vi "Test Communication.vi"() -> ()   [LabVIEW 2025]
uses:
  f24cd2ec-823b-4f95-a374-4134a1dae946.vi
  362e8ed5-b5fe-4805-bc07-5d5cfe9ff187.vi
  c76493dc-2eb4-4e37-bcd2-fc06ee71f938.vi
  523c6d7b-34c9-4a1f-add0-cf9b8ecace1d.vi
  a9163a1a-bf7f-4ec5-a553-ba6517dc0e79.vi
  6f03f4ed-4b4c-4e8a-979c-720ab53ff51f.vi
  PCAN2023/PCAN API.lvlib
  77574cea-78a9-48c4-8703-67bd64e21fec.vi
panel:
  in  "x":bool
  out "Numeric":i32
  out "MessageBuffer out 2":T1 {"ID" format="%.0x"}
  out "Boolean 2":bool
  out "Boolean":bool
  out "MessageBuffer out":T1 {"ID" format="%.0x"}
  out "error out":errorcluster
  in  "error in":errorcluster
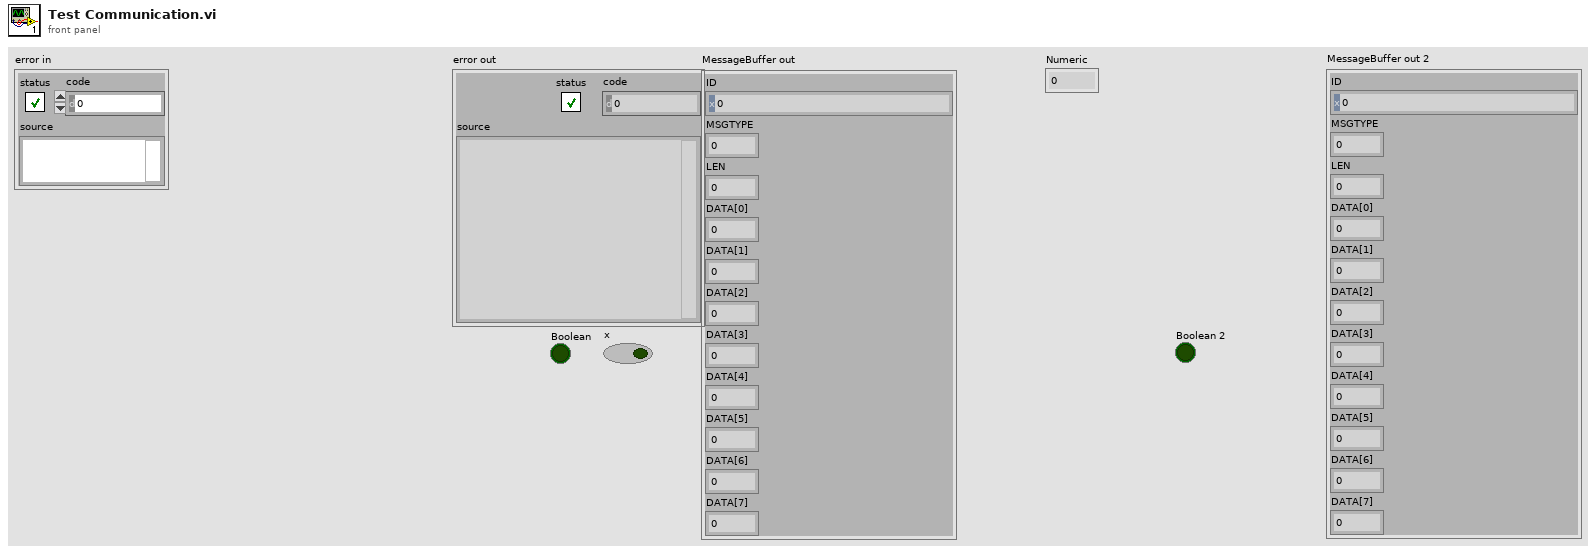
[diagram p1: front panel]
types:
  T1 = cluster{"ID":u32, "MSGTYPE":u8, "LEN":u8, "DATA[0]":u8, "DATA[1]":u8, "DATA[2]":u8, "DATA[3]":u8, "DATA[4]":u8, "DATA[5]":u8, "DATA[6]":u8, "DATA[7]":u8}
  T2 = cluster{"ID":u32, "MSGTYPE":u8, "DLC":u8, "DATA[0]":u8, "DATA[1]":u8, "DATA[2]":u8, "DATA[3]":u8, "DATA[4]":u8, "DATA[5]":u8, "DATA[6]":u8, "DATA[7]":u8, "DATA[8]":u8, "DATA[9]":u8, "DATA[10]":u8, "DATA[11]":u8, "DATA[12]":u8, "DATA[13]":u8, "DATA[14]":u8, "DATA[15]":u8, "DATA[16]":u8, "DATA[17]":u8, "DATA[18]":u8, "DATA[19]":u8, "DATA[20]":u8, "DATA[21]":u8, "DATA[22]":u8, "DATA[23]":u8, "DATA[24]":u8, "DATA[25]":u8, "DATA[26]":u8, "DATA[27]":u8, "DATA[28]":u8, "DATA[29]":u8, "DATA[30]":u8, "DATA[31]":u8, "DATA[32]":u8, "DATA[33]":u8, "DATA[34]":u8, "DATA[35]":u8, "DATA[36]":u8, "DATA[37]":u8, "DATA[38]":u8, "DATA[39]":u8, "DATA[40]":u8, "DATA[41]":u8, "DATA[42]":u8, "DATA[43]":u8, "DATA[44]":u8, "DATA[45]":u8, "DATA[46]":u8, "DATA[47]":u8, "DATA[48]":u8, "DATA[49]":u8, "DATA[50]":u8, "DATA[51]":u8, "DATA[52]":u8, "DATA[53]":u8, "DATA[54]":u8, "DATA[55]":u8, "DATA[56]":u8, "DATA[57]":u8, "DATA[58]":u8, "DATA[59]":u8, "DATA[60]":u8, "DATA[61]":u8, "DATA[62]":u8, "DATA[63]":u8}
  T3 = cluster{"ID":u32, "MSGTYPE":u8, "LEN":u8, "DATA[0]":u8, "DATA[1]":u8, "DATA[2]":u8, "DATA[3]":u8, "DATA[4]":u8, "DATA[5]":u8, "DATA[6]":u8, "DATA[7]":u8}[]
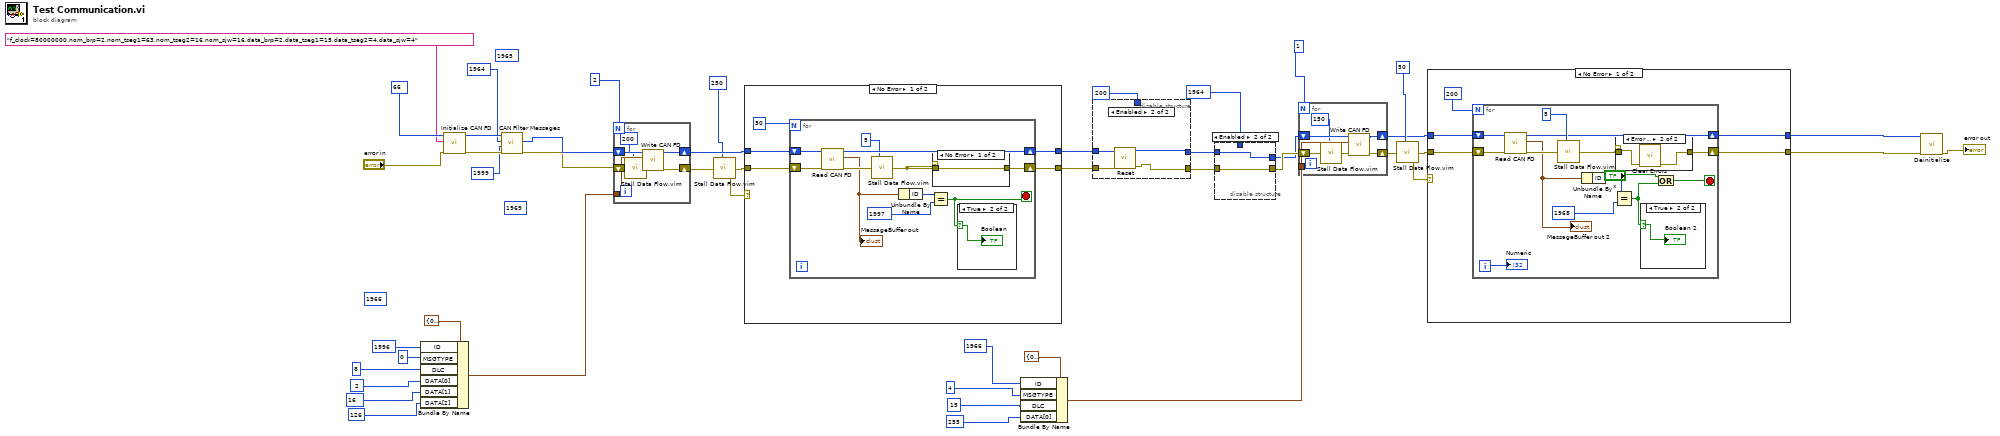
[diagram p0: block diagram]
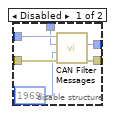
[diagram p2: hidden frame]
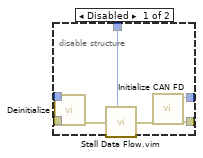
[diagram p3: hidden frame]
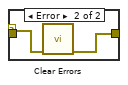
[diagram p4: hidden frame]
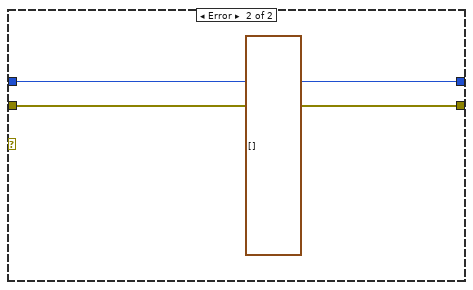
[diagram p6: hidden frame]
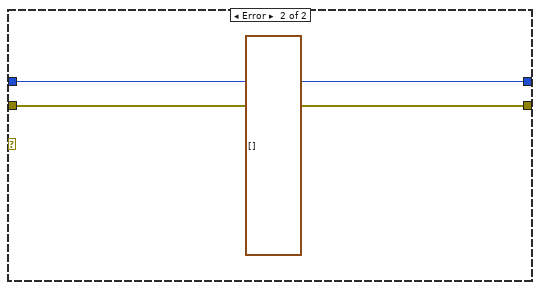
[diagram p9: hidden frame]
diagram:
  (unwired) u32 1969 ("FromID")
  (unwired) u32 1965 ("FromID")
  (unwired) u32 1966 ("ID")
  n1 = Bundle By Name(cluster=T2 {"ID"=0, "MSGTYPE"=0, "DLC"=0, "DATA[0]"=0, "DATA[1]"=0, "DATA[2]"=0, "DATA[3]"=0, "DATA[4]"=0, "DATA[5]"=0, "DATA[6]"=0, "DATA[7]"=0, "DATA[8]"=0, "DATA[9]"=0, "DATA[10]"=0, "DATA[11]"=0, "DATA[12]"=0, "DATA[13]"=0, "DATA[14]"=0, "DATA[15]"=0, "DATA[16]"=0, "DATA[17]"=0, "DATA[18]"=0, "DATA[19]"=0, "DATA[20]"=0, "DATA[21]"=0, "DATA[22]"=0, "DATA[23]"=0, "DATA[24]"=0, "DATA[25]"=0, "DATA[26]"=0, "DATA[27]"=0, "DATA[28]"=0, "DATA[29]"=0, "DATA[30]"=0, "DATA[31]"=0, "DATA[32]"=0, "DATA[33]"=0, "DATA[34]"=0, "DATA[35]"=0, "DATA[36]"=0, "DATA[37]"=0, "DATA[38]"=0, "DATA[39]"=0, "DATA[40]"=0, "DATA[41]"=0, "DATA[42]"=0, "DATA[43]"=0, "DATA[44]"=0, "DATA[45]"=0, "DATA[46]"=0, "DATA[47]"=0, "DATA[48]"=0, "DATA[49]"=0, "DATA[50]"=0, "DATA[51]"=0, "DATA[52]"=0, "DATA[53]"=0, "DATA[54]"=0, "DATA[55]"=0, "DATA[56]"=0, "DATA[57]"=0, "DATA[58]"=0, "DATA[59]"=0, "DATA[60]"=0, "DATA[61]"=0, "DATA[62]"=0, "DATA[63]"=0} ("MessageBuffer"), "ID"=u32 1996, "MSGTYPE"=u8 0, "DLC"=u8 8, "DATA[0]"=u8 2, "DATA[1]"=u8 16 ("DATA[0]"), "DATA[2]"=u8 126 ("DATA[0]")) -> (w40:T2)
  n2 = call "Initialize CAN FD.vi"("error in"="error in", "BitrateFD"="f_clock=80000000,nom_brp=2,nom_tseg1=63,nom_tseg2=16,nom_sjw=16,data_brp=2,data_tseg1=15,data_tseg2=4,data_sjw=4", "Channel"=u16 66) -> ("error out"=w33:errorcluster, "Channel out"=w34:u16)  [unwired: 7 in]
  n3 = call "CAN Filter Messages.vi"("error in (no error)"=w33, "ToID"=u32 1999 ("FromID"), "FromID"=u32 1964, "Channel in"=w34) -> ("error out"=w14:errorcluster, "Channel out"=w15:u16)  [unwired: 5 in, 1 out]
  n4 = for {
    N: 2 -> [_]
    tunnel: w40 -> [w49]
    shift-right: [w48] -> w13
    shift-left: w15 -> [w51]
    shift-right: [w47] -> w12
    shift-left: w14 -> [w50]
    n5 = call "Stall Data Flow.vim"("value in"=w50, "milliseconds to wait"=u32 200) -> ("value out"=w46:errorcluster)  [unwired: 1 out]
    n6 = call "Write CAN FD.vi"("error in (no error)"=w46, "MessageBuffer"=w49, "Channel"=w51) -> ("error out"=w47:errorcluster, "Channel out"=w48:u16)  [unwired: 7 in]
  }
  n7 = call "Stall Data Flow.vim"("value in"=w12, "milliseconds to wait"=u32 250) -> ("value out"=w10:errorcluster)  [unwired: 1 out]
  n8 = case shown="No Error" w10 {
    tunnel: w13 -> [w56 w73]
    tunnel: w10 -> [w55 w72]
    tunnel: [w54 w73] -> w8
    tunnel: [w53 w72] -> w7
    frame No Error {
      n9 = for {
        N: 50 -> [_]
        shift-right: [w63] -> w54
        shift-left: w56 -> [w64]
        shift-right: [w65] -> w53
        shift-left: w55 -> [w62]
        stop <- w59 stop-if-true
        n10 = call "Read CAN FD.vi"("error in"=w62, "Channel"=w64) -> ("error out"=w61:errorcluster, "MessageBuffer out"=w60:T1, "Channel out"=w63:u16)  [unwired: 7 in]
        "MessageBuffer out" <- w60
        n11 = call "Stall Data Flow.vim"("value in"=w61, "milliseconds to wait"=u32 5) -> ("value out"=w58:errorcluster)  [unwired: 1 out]
        n12 = Unbundle By Name(w60) -> ("ID"=w67:u32)
        n13 = Equal?(x=w67, y=u32 1997) -> (x = y?=w59:bool)
        n14 = case shown="No Error" w58 {
          selector: w58 -> [w68 w70]
          tunnel: w58 -> [_ _]
          tunnel: [w68 w69] -> w65
          frame No Error {
          }
          frame Error {
            n15 = call <vilib>:"Clear Errors.vi"("error in (no error)"=w70) -> ("error out"=w69:errorcluster)  [unwired: 5 in, 1 out]
          }
        }
        n16 = case shown="True" w59 {
          selector: w59 -> [_ w71]
          frame False {
          }
          frame True {
            "Boolean" <- w71
          }
        }
      }
    }
    frame Error {
      (unwired) T3 []
    }
  }
  n17 = Bundle By Name(cluster=T2 {"ID"=0, "MSGTYPE"=0, "DLC"=0, "DATA[0]"=0, "DATA[1]"=0, "DATA[2]"=0, "DATA[3]"=0, "DATA[4]"=0, "DATA[5]"=0, "DATA[6]"=0, "DATA[7]"=0, "DATA[8]"=0, "DATA[9]"=0, "DATA[10]"=0, "DATA[11]"=0, "DATA[12]"=0, "DATA[13]"=0, "DATA[14]"=0, "DATA[15]"=0, "DATA[16]"=0, "DATA[17]"=0, "DATA[18]"=0, "DATA[19]"=0, "DATA[20]"=0, "DATA[21]"=0, "DATA[22]"=0, "DATA[23]"=0, "DATA[24]"=0, "DATA[25]"=0, "DATA[26]"=0, "DATA[27]"=0, "DATA[28]"=0, "DATA[29]"=0, "DATA[30]"=0, "DATA[31]"=0, "DATA[32]"=0, "DATA[33]"=0, "DATA[34]"=0, "DATA[35]"=0, "DATA[36]"=0, "DATA[37]"=0, "DATA[38]"=0, "DATA[39]"=0, "DATA[40]"=0, "DATA[41]"=0, "DATA[42]"=0, "DATA[43]"=0, "DATA[44]"=0, "DATA[45]"=0, "DATA[46]"=0, "DATA[47]"=0, "DATA[48]"=0, "DATA[49]"=0, "DATA[50]"=0, "DATA[51]"=0, "DATA[52]"=0, "DATA[53]"=0, "DATA[54]"=0, "DATA[55]"=0, "DATA[56]"=0, "DATA[57]"=0, "DATA[58]"=0, "DATA[59]"=0, "DATA[60]"=0, "DATA[61]"=0, "DATA[62]"=0, "DATA[63]"=0} ("MessageBuffer"), "ID"=u32 1966, "MSGTYPE"=u8 4, "DLC"=u8 15, "DATA[0]"=u8 255) -> (w26:T2)
  n18 = disable-structure shown="Enabled" {
    disable-tunnel: w8 -> [w80 w84]
    disable-tunnel: w7 -> [w79 w83]
    disable-tunnel: [w78 w82] -> w6
    disable-tunnel: [w76 w81] -> w5
    disable-tunnel: u32 200 ("milliseconds to wait") -> [w74 _]
    frame Disabled {
      n19 = call "Deinitialize.vi"("error in"=w79, "Channel"=w80) -> ("error out"=w77:errorcluster)  [unwired: 9 in]
      n20 = call "Stall Data Flow.vim"("value in"=w77, "milliseconds to wait"=w74) -> ("value out"=w75:errorcluster)  [unwired: 1 out]
      n21 = call "Initialize CAN FD.vi"("error in"=w75) -> ("error out"=w76:errorcluster, "Channel out"=w78:u16)  [unwired: 9 in]
    }
    frame Enabled {
      n22 = call "Reset.vi"("error in"=w83, "Channel"=w84) -> ("error out"=w81:errorcluster, "Channel out"=w82:u16)  [unwired: 8 in]
    }
  }
  n23 = disable-structure shown="Enabled" {
    disable-tunnel: w6 -> [w90 w91]
    disable-tunnel: w5 -> [w89 w92]
    disable-tunnel: [w88 w92] -> w4
    disable-tunnel: [w87 w91] -> w3
    disable-tunnel: u32 1964 ("FromID") -> [w86 _]
    frame Disabled {
      n24 = call "CAN Filter Messages.vi"("error in (no error)"=w89, "ToID"=u32 1969 ("FromID"), "FromID"=w86, "Channel in"=w90) -> ("error out"=w88:errorcluster, "Channel out"=w87:u16)  [unwired: 5 in, 1 out]
    }
    frame Enabled {
    }
  }
  n25 = for {
    N: 1 -> [_]
    tunnel: w26 -> [w97]
    shift-right: [w96] -> w23
    shift-left: w3 -> [w99]
    shift-right: [w95] -> w22
    shift-left: w4 -> [w98]
    n26 = call "Stall Data Flow.vim"("value in"=w98, "milliseconds to wait"=u32 150) -> ("value out"=w94:errorcluster)  [unwired: 1 out]
    n27 = call "Write CAN FD.vi"("error in (no error)"=w94, "MessageBuffer"=w97, "Channel"=w99) -> ("error out"=w95:errorcluster, "Channel out"=w96:u16)  [unwired: 7 in]
  }
  n28 = call "Stall Data Flow.vim"("value in"=w22, "milliseconds to wait"=u32 50) -> ("value out"=w24:errorcluster)  [unwired: 1 out]
  n29 = case shown="No Error" w24 {
    tunnel: w23 -> [w104 w124]
    tunnel: w24 -> [w103 w123]
    tunnel: [w102 w124] -> w21
    tunnel: [w101 w123] -> w20
    frame No Error {
      n30 = for {
        N: 200 -> [_]
        shift-right: [w113] -> w102
        shift-left: w104 -> [w114]
        shift-right: [w116] -> w101
        shift-left: w103 -> [w112]
        i -> [w109]
        stop <- w106 stop-if-true
        n31 = call "Read CAN FD.vi"("error in"=w112, "Channel"=w114) -> ("error out"=w111:errorcluster, "MessageBuffer out"=w105:T1, "Channel out"=w113:u16)  [unwired: 7 in]
        "MessageBuffer out 2" <- w105
        n32 = call "Stall Data Flow.vim"("value in"=w111, "milliseconds to wait"=u32 5) -> ("value out"=w115:errorcluster)  [unwired: 1 out]
        n33 = Unbundle By Name(w105) -> ("ID"=w110:u32)
        n34 = Equal?(x=w110, y=u32 1968) -> (x = y?=w108:bool)
        n35 = case shown="Error .." w115 {
          selector: w115 -> [w119 w121]
          tunnel: w115 -> [_ _]
          tunnel: [w119 w120] -> w116
          frame No Error {
          }
          frame Error {
            n36 = call <vilib>:"Clear Errors.vi"("error in (no error)"=w121) -> ("error out"=w120:errorcluster)  [unwired: 5 in, 1 out]
          }
        }
        n37 = case shown="True" w108 {
          selector: w108 -> [_ w122]
          frame False {
          }
          frame True {
            "Boolean 2" <- w122
          }
        }
        n38 = Or(x="x", y=w108) -> (x .or. y?=w106:bool)
        "Numeric" <- w109
      }
    }
    frame Error {
      (unwired) T3 []
    }
  }
  n39 = call "Deinitialize.vi"("error in"=w20, "Channel"=w21) -> ("error out"=→"error out":errorcluster)  [unwired: 9 in]
